vi "EngineSim.vi"() -> ()   [LabVIEW 2013]
uses:
  Typedefs/PWM.ctl
  <vilib>/NI/Engine Simulation Toolkit (EST)/APU/Settings.ctl
  <vilib>/NI/Engine Simulation Toolkit (EST)/APU/Input.ctl
  <vilib>/NI/Engine Simulation Toolkit (EST)/APU/Output.ctl
  <vilib>/NI/Engine Simulation Toolkit (EST)/ECU Event/Timing/Capture Output.ctl
  <vilib>/NI/Engine Simulation Toolkit (EST)/ECU Event/Timing/Measure Settings.ctl
  <vilib>/NI/Engine Simulation Toolkit (EST)/ECU Event/Timing/Measure Output.ctl
  <vilib>/NI/Engine Simulation Toolkit (EST)/Digital Pattern Generation/Settings.ctl
  <vilib>/NI/Engine Simulation Toolkit (EST)/Digital Pattern Generation/Input.ctl
  <vilib>/NI/Engine Simulation Toolkit (EST)/Digital Pattern Generation/Load Input.ctl
  <vilib>/NI/Engine Simulation Toolkit (EST)/Knock Sensor/Cylinder Input.ctl
  <vilib>/NI/Engine Simulation Toolkit (EST)/Knock Sensor/Cylinder Settings.ctl
  <vilib>/NI/Engine Simulation Toolkit (EST)/Knock Sensor/Generate Input.ctl
  <vilib>/NI/Engine Simulation Toolkit (EST)/Knock Sensor/Generate Settings.ctl
  <vilib>/NI/Engine Simulation Toolkit (EST)/Version Token.ctl
  <vilib>/NI/Engine Simulation Toolkit (EST)/APU/Shared Settings.ctl
  <vilib>/Platform/TimedLoop/XDataNode/timing_clust.ctl
  <vilib>/Platform/TimedLoop/XDataNode/nitl_modes.ctl
  <vilib>/Platform/TimedLoop/XDataNode/wakeup.ctl
  <vilib>/NI/Engine Simulation Toolkit (EST)/ECU Event/Timing/Capture Settings.ctl
  <vilib>/rvi/DataTransferAndStorage/Container/Common/niFpgaContainerGetUniqueNameForEmu.vi
  <vilib>/rvi/DataTransferAndStorage/Container/Common/niFpgaContainerSetEmuInfo.vi
  <vilib>/rvi/eio/common/nirviEmuReportErrorAndStop.vi
  <vilib>/rvi/Emulation/niFpgaSctlEmulationGetInTimedLoop.vi
  <vilib>/rvi/Emulation/niFpgaEmulationReportErrorSimple.vi
  <vilib>/rvi/Emulation/niFpgaGetClockAttributes.vi
  <vilib>/rvi/Emulation/niFpgaCriticalErrorInLSC.vi
  <vilib>/rvi/eio/common/nirviEmuTemplateMethod_errors.vi
  <vilib>/NI/Engine Simulation Toolkit (EST)/ECU Event/Timing/Measure Events (Non-40MHz).vi
  <vilib>/Platform/TimedLoop/XDataNode/XDataNode.xnode
  <vilib>/rvi/LocalResourceManager/LocalResourceManager.xnode
  <vilib>/eio/EIONode/EIONode.xnode
  <vilib>/Platform/TimedLoop/XDataNode/XDNodeRunTimeDep.lvlib
  <vilib>/NI/Engine Simulation Toolkit (EST)/APU/APU.lvlib
  <vilib>/NI/Engine Simulation Toolkit (EST)/ECU Event/Timing/ECU Event Timing.lvlib
  <vilib>/NI/Engine Simulation Toolkit (EST)/Digital Pattern Generation/Digital Pattern Generation.lvlib
  <vilib>/NI/Engine Simulation Toolkit (EST)/Knock Sensor/Knock Sensor.lvlib
  <vilib>/NI/Engine Simulation Toolkit (EST)/Engine Simulation Toolkit.lvlib
panel:
  in  "shared settings.apu":T1 {"cycle start" format="%#.15g"}
  in  "go.apu":bool
  in  "Spark Filter Ticks":fxp<+,11,11>=350.0
  in  "Injector Filter Ticks":fxp<+,11,11>=100.0
  in  "est.version":T2
  in  "settings.Knock AO 2":T3
  in  "settings.Knock AO 2.Cylinder 1":T4
  in  "settings.Knock AO 2.Cylinder 2":T4
  in  "settings.Knock AO 2.Cylinder 3":T4
  in  "settings.Knock AO 2.Cylinder 4":T4
  in  "input.Knock AO 2.Cylinder 1":T5
  in  "input.Knock AO 2.Cylinder 2":T5
  in  "input.Knock AO 2.Cylinder 3":T5
  in  "input.Knock AO 2.Cylinder 4":T5
  in  "input.Knock AO 2":T6
  in  "settings.Knock AO 2.Cylinder 5":T4
  in  "settings.Knock AO 2.Cylinder 6":T4
  in  "input.Knock AO 2.Cylinder 5":T5
  in  "input.Knock AO 2.Cylinder 6":T5
  in  "load input.Cam":T7
  in  "load input.Crank":T7
  in  "input.Crank":T8
  in  "settings.Crank":T9
  in  "input.Cam":T8
  in  "settings.Cam":T9
  out "status.Fuel6":T10
  in  "settings.Fuel6":T11
  out "capture.Fuel6.event 1":T12
  out "status.Fuel5":T10
  in  "settings.Fuel5":T11
  out "capture.Fuel5.event 1":T12
  out "status.Fuel4":T10
  in  "settings.Fuel4":T11
  out "capture.Fuel4.event 1":T12
  out "status.Fuel3":T10
  in  "settings.Fuel3":T11
  out "capture.Fuel3.event 1":T12
  out "status.Fuel2":T10
  in  "settings.Fuel2":T11
  out "capture.Fuel2.event 1":T12
  out "status.Fuel1":T10
  in  "settings.Fuel1":T11
  out "capture.Fuel1.event 1":T12
  out "status.Spark6":T10
  in  "settings.Spark6":T11
  out "capture.Spark6.event 1":T12
  out "status.Spark5":T10
  in  "settings.Spark5":T11
  out "capture.Spark5.event 1":T12
  out "status.Spark4":T10
  in  "settings.Spark4":T11
  out "capture.Spark4.event 1":T12
  out "status.Spark3":T10
  in  "settings.Spark3":T11
  out "capture.Spark3.event 1":T12
  out "status.Spark2":T10
  in  "settings.Spark2":T11
  out "capture.Spark2.event 1":T12
  out "status.Spark1":T10
  in  "settings.Spark1":T11
  out "capture.Spark1.event 1":T12
  out "output.apu":T13 caption="output"
  in  "input.apu":T14 caption="input"
  in  "settings.apu":T15
  in  "PWM write.Key Switch":T16
  in  "PWM write.Airflow":T16
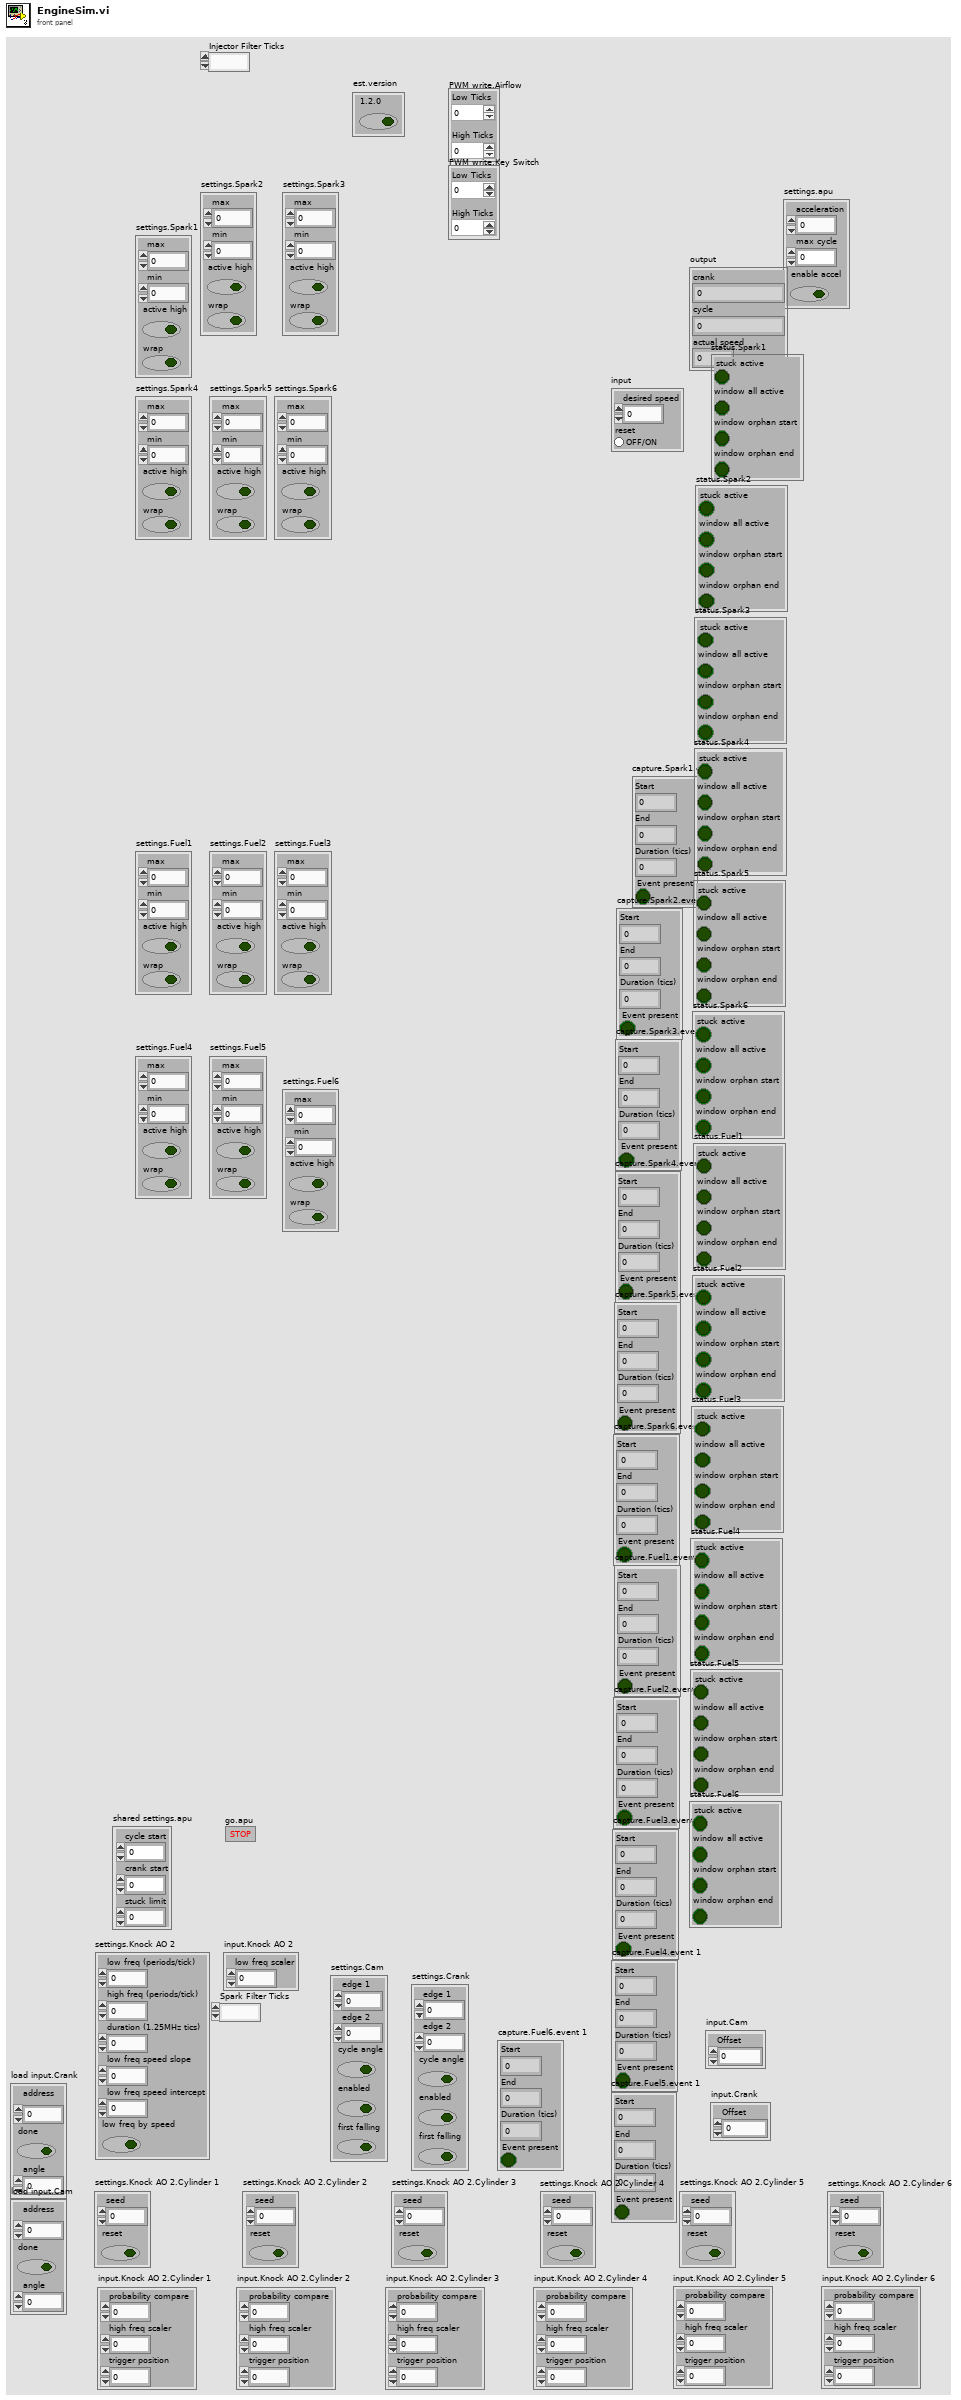
[diagram p1: front panel]
types:
  T1 = typedef "Engine Simulation Toolkit.lvlib/APU.lvlib/Shared Settings.ctl" = cluster{"cycle start":fxp<+,2,2>, "crank start":u16, "stuck limit":fxp<+,18,18>}
  T2 = typedef "Engine Simulation Toolkit.lvlib/Version Token.ctl" = cluster{"1.2.0":bool}
  T3 = typedef "Engine Simulation Toolkit.lvlib/Knock Sensor.lvlib/Generate Settings.ctl" = cluster{"low freq (periods/tick)":fxp<+,32,0>, "high freq (periods/tick)":fxp<+,32,0>, "duration (1.25MHz tics)":fxp<+,18,18>, "low freq speed slope":fxp<+,16,-3>, "low freq speed intercept":fxp<+,10,-10>, "low freq by speed":bool}
  T4 = typedef "Engine Simulation Toolkit.lvlib/Knock Sensor.lvlib/Cylinder Settings.ctl" = cluster{"seed":u16, "reset":bool}
  T5 = typedef "Engine Simulation Toolkit.lvlib/Knock Sensor.lvlib/Cylinder Input.ctl" = cluster{"probability compare":u16, "high freq scaler":fxp<+,10,0>, "trigger position":u16}
  T6 = typedef "Engine Simulation Toolkit.lvlib/Knock Sensor.lvlib/Generate Input.ctl" = cluster{"low freq scaler":fxp<+,10,0>}
  T7 = typedef "Engine Simulation Toolkit.lvlib/Digital Pattern Generation.lvlib/Load Input.ctl" = cluster{"address":fxp<+,11,11>, "done":bool, "angle":u16}
  T8 = typedef "Engine Simulation Toolkit.lvlib/Digital Pattern Generation.lvlib/Input.ctl" = cluster{"Offset":i16}
  T9 = typedef "Engine Simulation Toolkit.lvlib/Digital Pattern Generation.lvlib/Settings.ctl" = cluster{"edge 1":u16, "edge 2":u16, "cycle angle":bool, "enabled":bool, "first falling":bool}
  T10 = typedef "Engine Simulation Toolkit.lvlib/ECU Event Timing.lvlib/Measure Output.ctl" = cluster{"stuck active":bool, "window all active":bool, "window orphan start":bool, "window orphan end":bool}
  T11 = typedef "Engine Simulation Toolkit.lvlib/ECU Event Timing.lvlib/Measure Settings.ctl" = cluster{"max":u16, "min":u16, "active high":bool, "wrap":bool}
  T12 = typedef "Engine Simulation Toolkit.lvlib/ECU Event Timing.lvlib/Capture Output.ctl" = cluster{"Start":u16, "End":u16, "Duration (tics)":fxp<+,18,18>, "Event present":bool}
  T13 = typedef "Engine Simulation Toolkit.lvlib/APU.lvlib/Output.ctl" = cluster{"crank":u16, "cycle":u16, "actual speed":fxp<+/-,23,2>}
  T14 = typedef "Engine Simulation Toolkit.lvlib/APU.lvlib/Input.ctl" = cluster{"desired speed":fxp<+/-,23,2>, "reset":bool}
  T15 = typedef "Engine Simulation Toolkit.lvlib/APU.lvlib/Settings.ctl" = cluster{"acceleration":fxp<+,18,-20>, "max cycle":fxp<+,2,2>, "enable accel":bool}
  T16 = typedef "PWM.ctl" = cluster{"Low Ticks":u32, "High Ticks":u32}
  T17 = typedef "XDNodeRunTimeDep.lvlib/timing_clust.ctl" = cluster{"Expected End [f-1]":u64, "Actual End [f-1]":u64, "Finished Late? [f-1]":bool, "Expected End [i-1]":u64, "Actual End [i-1]":u64, "Finished Late? [i-1]":bool, "Expected Start [i]":u64, "Actual Start [i]":u64, "Expected Start [f]":u64, "Actual Start [f]":u64, "Source Name":string, "Structure Name":string, "Period":i64, "Deadline":i64, "Offset":i64, "Start":i64, "Priority":i32, "Timeout":i32, "Mode":T18, "Wakeup Reason":T19, "Error":errorcluster, "Source Type":string, "Secondary Source Type":string, "Global End Time":u64, "Global Start Time":u64, "Frame Duration":u64, "Iteration Duration":u64, "Assigned CPU":i32, "I/O Scan Engine Mode":u32}
  T18 = typedef "XDNodeRunTimeDep.lvlib/nitl_modes.ctl" = enum32{"No Change", "Process missed periods, maintain original phase", "Discard missed periods, maintain original phase", "Process missed periods, ignore original phase", "Discard missed periods, ignore original phase"}
  T19 = typedef "XDNodeRunTimeDep.lvlib/wakeup.ctl" = enum32{"Normal", "Aborted", "Asynchronous wakeup", "Timing source error", "Timed loop error", "Timeout"}
  T20 = typedef "Engine Simulation Toolkit.lvlib/Digital Pattern Generation.lvlib/Load Data.ctl" = cluster{"max address":fxp<+,11,11>, "memory":refnum<k21>}
  T21 = typedef "Engine Simulation Toolkit.lvlib/APU.lvlib/Register Bus.ctl" = cluster{"Speed":refnum<k21>, "Crank Angle":refnum<k21>, "Cycle Angle":refnum<k21>, "Crank Count":refnum<k21>, "Cycle Count":refnum<k21>, "1.25 MHz Counter":refnum<k21>, "shared settings":T1}
  T22 = typedef "Engine Simulation Toolkit.lvlib/ECU Event Timing.lvlib/Capture Settings.ctl" = u8
  T23 = typedef "Engine Simulation Toolkit.lvlib/ECU Event Timing.lvlib/Measured Data.ctl" = cluster{"start":u16, "end":u16, "duration (tics)":fxp<+,18,18>, "window end":bool, "window begin":bool, "pulse end":bool, "pulse #":u8}
  T24 = typedef "Engine Simulation Toolkit.lvlib/Knock Sensor.lvlib/Triggered Cylinder Data.ctl" = cluster{"trigger knock":bool, "high freq scaler":fxp<+,10,0>}
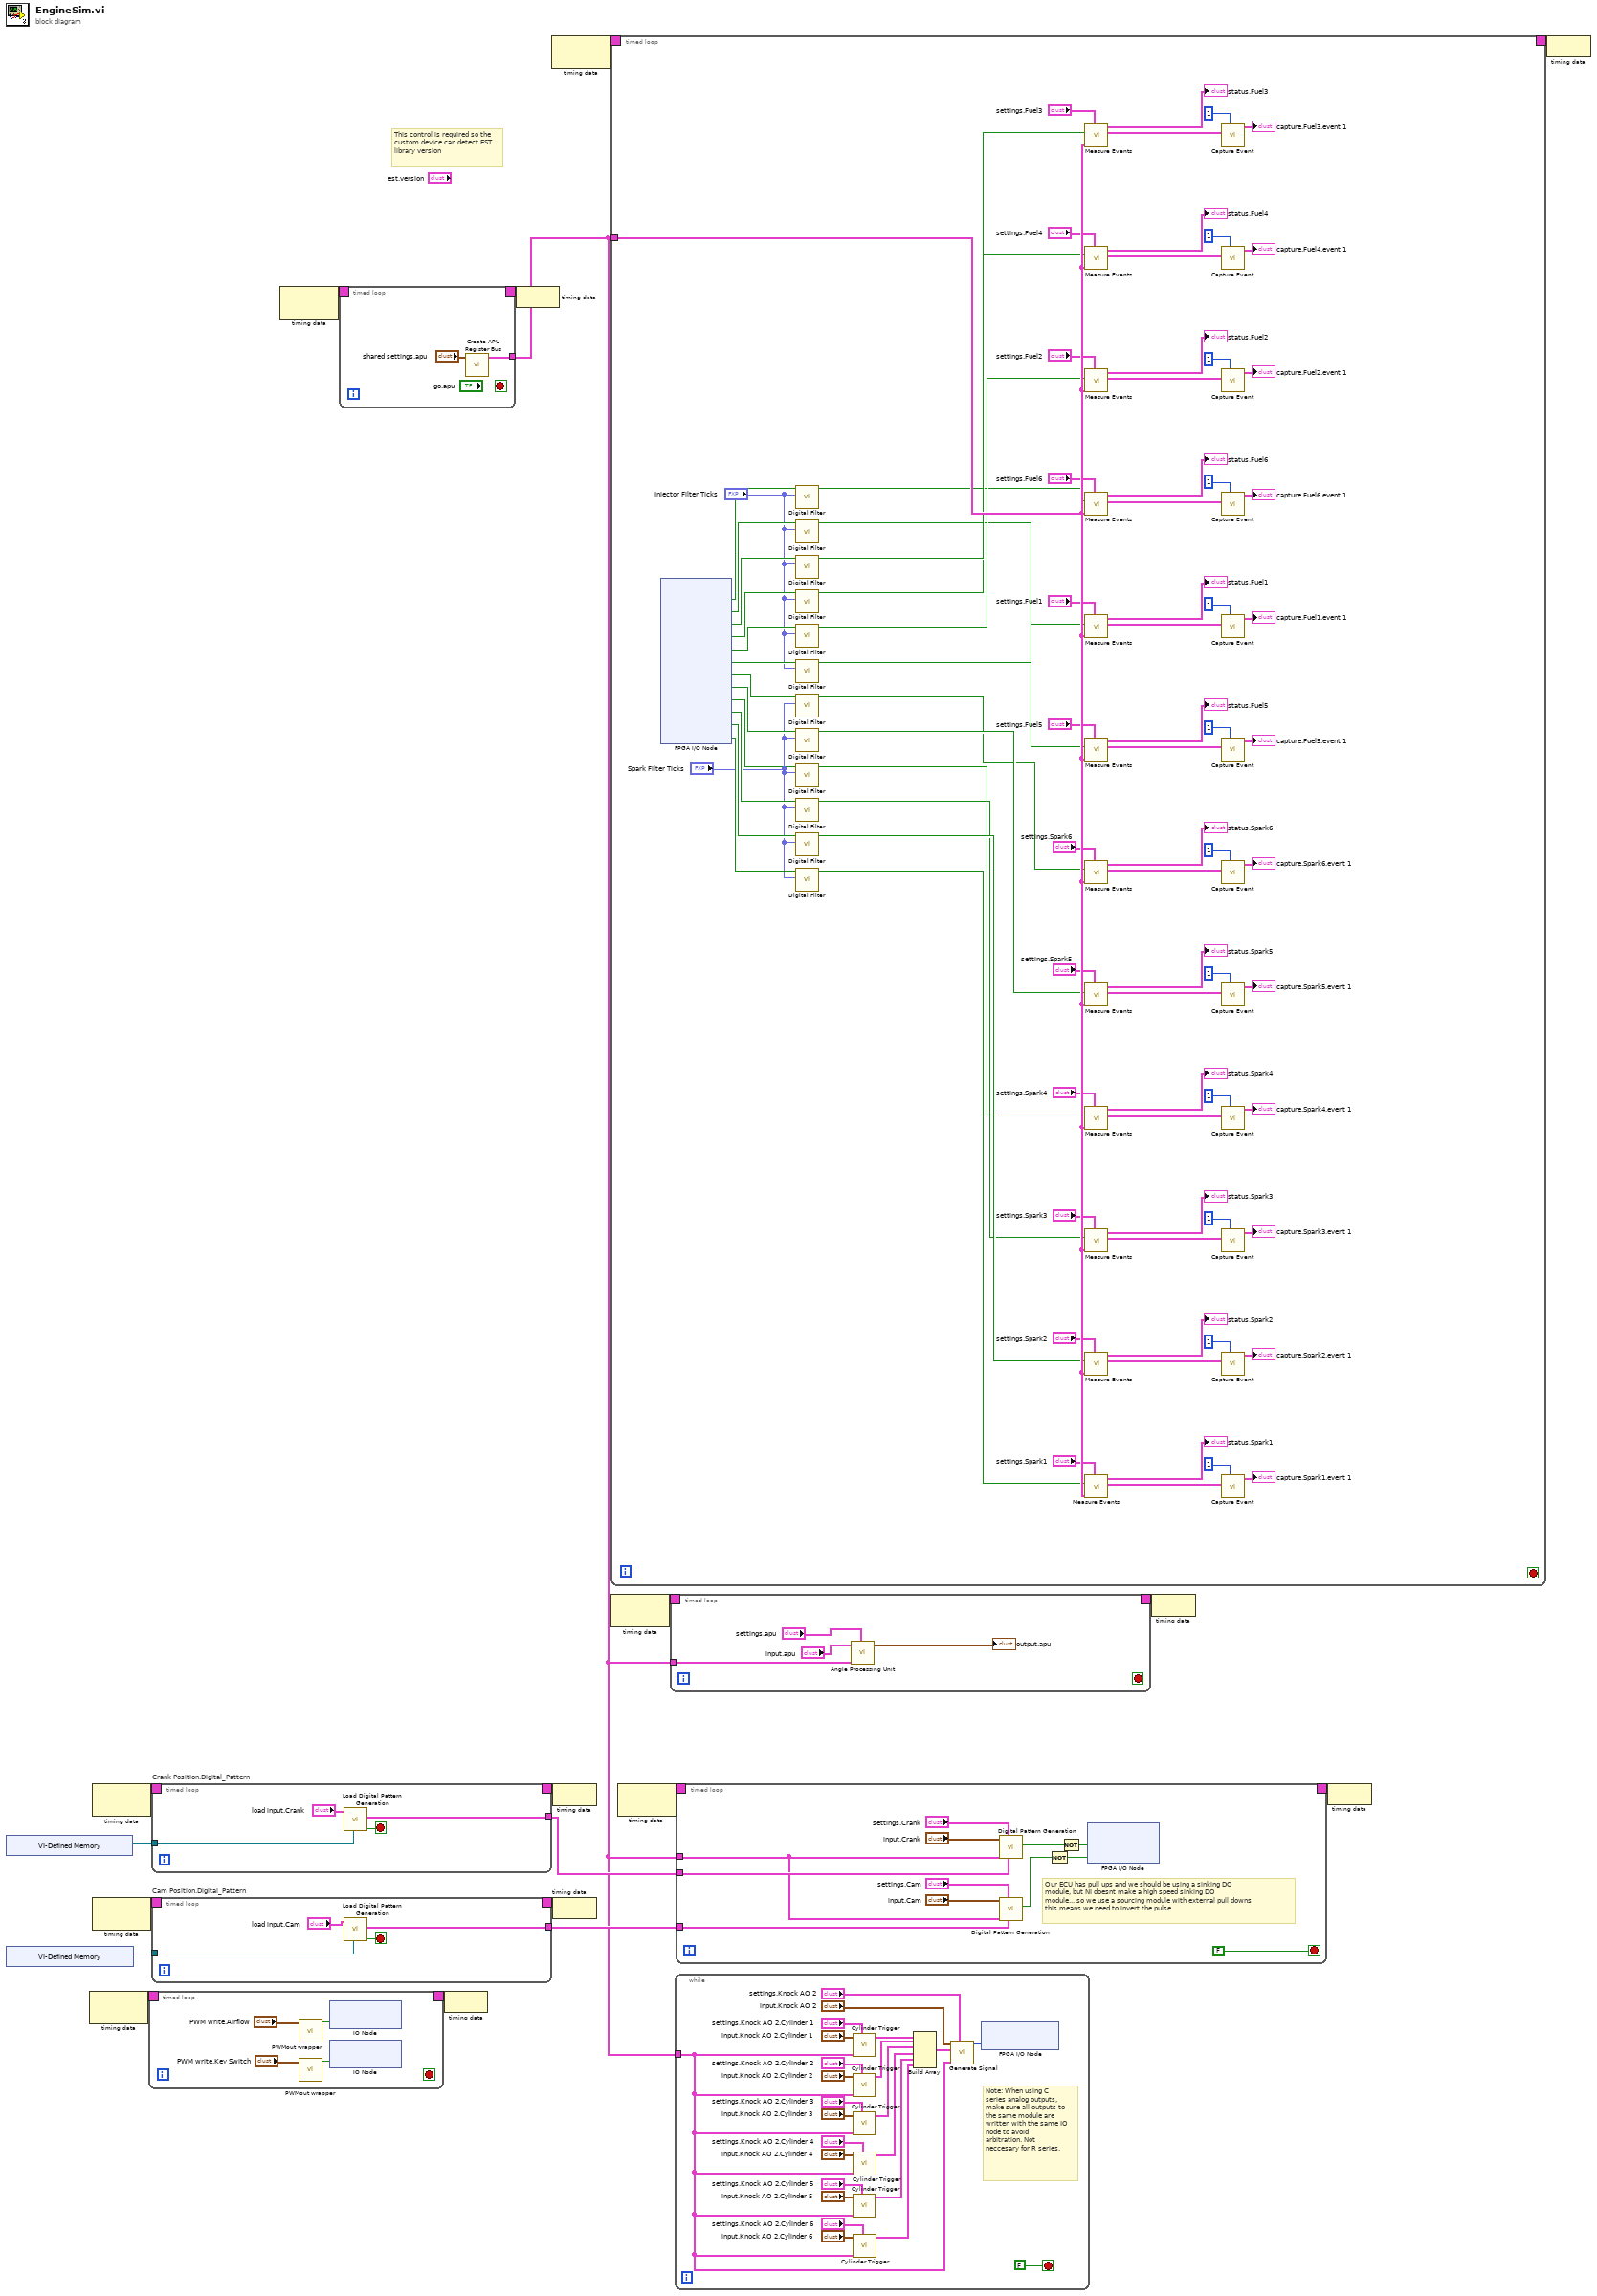
[diagram p0: block diagram]
diagram:
  # "This control is required so the custom device can detect EST library version"
  n1 = xnode "VI-Defined Memory"() -> ("Memory Out"=w7:refnum<k21>)
  n2 = xnode "VI-Defined Memory"() -> ("Memory Out"=w6:refnum<k21>)
  n3 = node-c288() -> (w19:T17)  [unwired: 1 in]
  n4 = node-c288() -> (w13:T17)  [unwired: 1 in]
  n5 = node-c288() -> (w11:T17)  [unwired: 1 in]
  n6 = timed-loop {
    timing: w19 -> [_]
    timing-out: [_] -> w18
    stop <- _ stop-if-true
    n7 = call "PWMout wrapper.vi"("PWM in"="PWM write.Airflow") -> ("Value"=w23:bool)  [unwired: 10 in]
    n8 = call "PWMout wrapper.vi"("PWM in"="PWM write.Key Switch") -> ("Value"=w21:bool)  [unwired: 10 in]
    n9 = xnode ("IO Node")("9474/DO3"=w23) -> ()  [unwired: 1 in, 1 out]
    n10 = xnode ("IO Node")("9474/DO4"=w21) -> ()  [unwired: 1 in, 1 out]
  }
  n11 = timed-loop "Crank Position.Digital_Pattern" {
    timing: w13 -> [_]
    timing-out: [_] -> w12
    tunnel: w7 -> [w28]
    tunnel: [w27] -> w9
    stop <- w29 stop-if-true
    n12 = call <vilib>:"Load Digital Pattern Generation.vi"("memory"=w28, "load input.<user name>"="load input.Crank") -> ("done"=w29:bool, "load data"=w27:T20)  [unwired: 8 in]
  }
  n13 = timed-loop "Cam Position.Digital_Pattern" {
    timing: w11 -> [_]
    timing-out: [_] -> w10
    tunnel: w6 -> [w34]
    tunnel: [w33] -> w8
    stop <- w35 stop-if-true
    n14 = call <vilib>:"Load Digital Pattern Generation.vi"("memory"=w34, "load input.<user name>"="load input.Cam") -> ("done"=w35:bool, "load data"=w33:T20)  [unwired: 8 in]
  }
  n15 = node-c288() -> (w3:T17)  [unwired: 1 in]
  n16 = timed-loop {
    timing: w3 -> [_]
    timing-out: [_] -> w2
    tunnel: [w39] -> w1
    stop <- "go.apu" stop-if-true
    n17 = call <vilib>:"Create APU Register Bus.vi"("shared settings.<user name>"="shared settings.apu") -> ("register bus"=w39:T21)  [unwired: 10 in]
  }
  n18 = node-c288(w18) -> ()
  n19 = node-c288(w2) -> ()
  n20 = node-c288() -> (w5:T17)  [unwired: 1 in]
  n21 = node-c288(w12) -> ()
  n22 = node-c288(w10) -> ()
  n23 = timed-loop "NI 9403" {
    tunnel: w1 -> [w129]
    timing: w5 -> [_]
    timing-out: [_] -> w4
    stop <- _ stop-if-true
    n24 = xnode "FPGA I/O Node"() -> ("Fuel/DI5"=w128:bool, "Fuel/DI4"=w127:bool, "Fuel/DI3"=w126:bool, "Fuel/DI2"=w125:bool, "Fuel/DI1"=w124:bool, "Fuel/DI0"=w123:bool, "Spark/DI5"=w122:bool, "Spark/DI4"=w121:bool, "Spark/DI3"=w120:bool, "Spark/DI2"=w119:bool, "Spark/DI1"=w118:bool, "Spark/DI0"=w117:bool)  [unwired: 12 in, 12 out]
    n25 = call "Digital Filter.vi"("Tics to Filter"="Injector Filter Ticks", "Input Signal"=w128) -> ("Output Filtered Signal"=w48:bool)  [unwired: 9 in]
    n26 = call "Digital Filter.vi"("Tics to Filter"="Injector Filter Ticks", "Input Signal"=w127) -> ("Output Filtered Signal"=w49:bool)  [unwired: 9 in]
    n27 = call "Digital Filter.vi"("Tics to Filter"="Injector Filter Ticks", "Input Signal"=w126) -> ("Output Filtered Signal"=w50:bool)  [unwired: 9 in]
    n28 = call "Digital Filter.vi"("Tics to Filter"="Injector Filter Ticks", "Input Signal"=w125) -> ("Output Filtered Signal"=w45:bool)  [unwired: 9 in]
    n29 = call "Digital Filter.vi"("Tics to Filter"="Injector Filter Ticks", "Input Signal"=w124) -> ("Output Filtered Signal"=w51:bool)  [unwired: 9 in]
    n30 = call "Digital Filter.vi"("Tics to Filter"="Injector Filter Ticks", "Input Signal"=w123) -> ("Output Filtered Signal"=w52:bool)  [unwired: 9 in]
    n31 = call "Digital Filter.vi"("Tics to Filter"="Spark Filter Ticks", "Input Signal"=w122) -> ("Output Filtered Signal"=w53:bool)  [unwired: 9 in]
    n32 = call "Digital Filter.vi"("Tics to Filter"="Spark Filter Ticks", "Input Signal"=w121) -> ("Output Filtered Signal"=w54:bool)  [unwired: 9 in]
    n33 = call "Digital Filter.vi"("Tics to Filter"="Spark Filter Ticks", "Input Signal"=w120) -> ("Output Filtered Signal"=w47:bool)  [unwired: 9 in]
    n34 = call "Digital Filter.vi"("Tics to Filter"="Spark Filter Ticks", "Input Signal"=w119) -> ("Output Filtered Signal"=w55:bool)  [unwired: 9 in]
    n35 = call "Digital Filter.vi"("Tics to Filter"="Spark Filter Ticks", "Input Signal"=w118) -> ("Output Filtered Signal"=w56:bool)  [unwired: 9 in]
    n36 = call "Digital Filter.vi"("Tics to Filter"="Spark Filter Ticks", "Input Signal"=w117) -> ("Output Filtered Signal"=w46:bool)  [unwired: 9 in]
    n37 = call-poly <vilib>:"Measure Events.vi"("settings.<user name>"="settings.Fuel3", "register bus"=w129, "event"=w45) -> ("measured data"=w73:T23, "status.<user name>"=→"status.Fuel3":T10)  [unwired: 7 in]
    n38 = call-poly <vilib>:"Measure Events.vi"("settings.<user name>"="settings.Fuel4", "register bus"=w129, "event"=w50) -> ("measured data"=w68:T23, "status.<user name>"=→"status.Fuel4":T10)  [unwired: 7 in]
    n39 = call-poly <vilib>:"Measure Events.vi"("settings.<user name>"="settings.Fuel2", "register bus"=w129, "event"=w51) -> ("measured data"=w78:T23, "status.<user name>"=→"status.Fuel2":T10)  [unwired: 7 in]
    n40 = call-poly <vilib>:"Measure Events.vi"("settings.<user name>"="settings.Fuel6", "register bus"=w129, "event"=w48) -> ("measured data"=w58:T23, "status.<user name>"=→"status.Fuel6":T10)  [unwired: 7 in]
    n41 = call-poly <vilib>:"Measure Events.vi"("settings.<user name>"="settings.Fuel1", "register bus"=w129, "event"=w52) -> ("measured data"=w83:T23, "status.<user name>"=→"status.Fuel1":T10)  [unwired: 7 in]
    n42 = call-poly <vilib>:"Measure Events.vi"("settings.<user name>"="settings.Fuel5", "register bus"=w129, "event"=w49) -> ("measured data"=w63:T23, "status.<user name>"=→"status.Fuel5":T10)  [unwired: 7 in]
    n43 = call-poly <vilib>:"Measure Events.vi"("settings.<user name>"="settings.Spark6", "register bus"=w129, "event"=w53) -> ("measured data"=w88:T23, "status.<user name>"=→"status.Spark6":T10)  [unwired: 7 in]
    n44 = call-poly <vilib>:"Measure Events.vi"("settings.<user name>"="settings.Spark5", "register bus"=w129, "event"=w54) -> ("measured data"=w93:T23, "status.<user name>"=→"status.Spark5":T10)  [unwired: 7 in]
    n45 = call-poly <vilib>:"Measure Events.vi"("settings.<user name>"="settings.Spark4", "register bus"=w129, "event"=w47) -> ("measured data"=w98:T23, "status.<user name>"=→"status.Spark4":T10)  [unwired: 7 in]
    n46 = call-poly <vilib>:"Measure Events.vi"("settings.<user name>"="settings.Spark3", "register bus"=w129, "event"=w55) -> ("measured data"=w103:T23, "status.<user name>"=→"status.Spark3":T10)  [unwired: 7 in]
    n47 = call-poly <vilib>:"Measure Events.vi"("settings.<user name>"="settings.Spark2", "register bus"=w129, "event"=w56) -> ("measured data"=w108:T23, "status.<user name>"=→"status.Spark2":T10)  [unwired: 7 in]
    n48 = call-poly <vilib>:"Measure Events.vi"("settings.<user name>"="settings.Spark1", "register bus"=w129, "event"=w46) -> ("measured data"=w113:T23, "status.<user name>"=→"status.Spark1":T10)  [unwired: 7 in]
    n49 = call <vilib>:"Capture Event.vi"("event # to capture"=T22 1 ("Settings.spark 1 shot 1"), "measured data"=w73) -> ("capture.<user name>"=→"capture.Fuel3.event 1":T12)  [unwired: 9 in]
    n50 = call <vilib>:"Capture Event.vi"("event # to capture"=T22 1 ("Settings.spark 1 shot 1"), "measured data"=w68) -> ("capture.<user name>"=→"capture.Fuel4.event 1":T12)  [unwired: 9 in]
    n51 = call <vilib>:"Capture Event.vi"("event # to capture"=T22 1 ("Settings.spark 1 shot 1"), "measured data"=w78) -> ("capture.<user name>"=→"capture.Fuel2.event 1":T12)  [unwired: 9 in]
    n52 = call <vilib>:"Capture Event.vi"("event # to capture"=T22 1 ("Settings.spark 1 shot 1"), "measured data"=w58) -> ("capture.<user name>"=→"capture.Fuel6.event 1":T12)  [unwired: 9 in]
    n53 = call <vilib>:"Capture Event.vi"("event # to capture"=T22 1 ("Settings.spark 1 shot 1"), "measured data"=w83) -> ("capture.<user name>"=→"capture.Fuel1.event 1":T12)  [unwired: 9 in]
    n54 = call <vilib>:"Capture Event.vi"("event # to capture"=T22 1 ("Settings.spark 1 shot 1"), "measured data"=w63) -> ("capture.<user name>"=→"capture.Fuel5.event 1":T12)  [unwired: 9 in]
    n55 = call <vilib>:"Capture Event.vi"("event # to capture"=T22 1 ("Settings.spark 1 shot 1"), "measured data"=w88) -> ("capture.<user name>"=→"capture.Spark6.event 1":T12)  [unwired: 9 in]
    n56 = call <vilib>:"Capture Event.vi"("event # to capture"=T22 1 ("Settings.spark 1 shot 1"), "measured data"=w93) -> ("capture.<user name>"=→"capture.Spark5.event 1":T12)  [unwired: 9 in]
    n57 = call <vilib>:"Capture Event.vi"("event # to capture"=T22 1 ("Settings.spark 1 shot 1"), "measured data"=w98) -> ("capture.<user name>"=→"capture.Spark4.event 1":T12)  [unwired: 9 in]
    n58 = call <vilib>:"Capture Event.vi"("event # to capture"=T22 1 ("Settings.spark 1 shot 1"), "measured data"=w103) -> ("capture.<user name>"=→"capture.Spark3.event 1":T12)  [unwired: 9 in]
    n59 = call <vilib>:"Capture Event.vi"("event # to capture"=T22 1 ("Settings.spark 1 shot 1"), "measured data"=w108) -> ("capture.<user name>"=→"capture.Spark2.event 1":T12)  [unwired: 9 in]
    n60 = call <vilib>:"Capture Event.vi"("event # to capture"=T22 1 ("Settings.spark 1 shot 1"), "measured data"=w113) -> ("capture.<user name>"=→"capture.Spark1.event 1":T12)  [unwired: 9 in]
  }
  n61 = node-c288() -> (w17:T17)  [unwired: 1 in]
  n62 = node-c288() -> (w15:T17)  [unwired: 1 in]
  n63 = timed-loop {
    timing: w17 -> [_]
    timing-out: [_] -> w16
    tunnel: w1 -> [w133]
    stop <- _ stop-if-true
    n64 = call <vilib>:"Angle Processing Unit.vi"("settings.<user name>"="settings.apu", "register bus"=w133, "input.<user name>"="input.apu") -> ("output.<user name>"=→"output.apu":T13)  [unwired: 8 in]
  }
  n65 = while {
    tunnel: w1 -> [w138]
    stop <- FALSE stop-if-true
    # "Note: When using C series analog outputs, make sure all outputs to the same module are written with the same IO node to avoid arbitration. Not neccesary for R series."
    n66 = call <vilib>:"Cylinder Trigger.vi"("settings.<user name>"="settings.Knock AO 2.Cylinder 1", "register bus"=w138, "input.<user name>"="input.Knock AO 2.Cylinder 1") -> ("triggered knock data"=w161:T24)  [unwired: 8 in]
    n67 = call <vilib>:"Cylinder Trigger.vi"("settings.<user name>"="settings.Knock AO 2.Cylinder 2", "register bus"=w138, "input.<user name>"="input.Knock AO 2.Cylinder 2") -> ("triggered knock data"=w160:T24)  [unwired: 8 in]
    n68 = call <vilib>:"Cylinder Trigger.vi"("settings.<user name>"="settings.Knock AO 2.Cylinder 3", "register bus"=w138, "input.<user name>"="input.Knock AO 2.Cylinder 3") -> ("triggered knock data"=w159:T24)  [unwired: 8 in]
    n69 = call <vilib>:"Cylinder Trigger.vi"("settings.<user name>"="settings.Knock AO 2.Cylinder 5", "register bus"=w138, "input.<user name>"="input.Knock AO 2.Cylinder 5") -> ("triggered knock data"=w140:T24)  [unwired: 8 in]
    n70 = call <vilib>:"Cylinder Trigger.vi"("settings.<user name>"="settings.Knock AO 2.Cylinder 4", "register bus"=w138, "input.<user name>"="input.Knock AO 2.Cylinder 4") -> ("triggered knock data"=w158:T24)  [unwired: 8 in]
    n71 = call <vilib>:"Cylinder Trigger.vi"("settings.<user name>"="settings.Knock AO 2.Cylinder 6", "register bus"=w138, "input.<user name>"="input.Knock AO 2.Cylinder 6") -> ("triggered knock data"=w139:T24)  [unwired: 8 in]
    n72 = Build Array(w161, w160, w159, w158, w140, w139) -> (w157:T24[])
    n73 = call <vilib>:"Generate Signal.vi"("settings.<user name>"="settings.Knock AO 2", "register bus"=w138, "triggered knock data"=w157, "input.<user name>"="input.Knock AO 2") -> ("knock signal"=w145:i16)  [unwired: 7 in]
    n74 = xnode ("FPGA I/O Node")("Knock/AO0"=w145) -> ()  [unwired: 1 in, 1 out]
  }
  n75 = timed-loop "Timed Loop" {
    timing: w15 -> [_]
    timing-out: [_] -> w14
    tunnel: w8 -> [w166]
    tunnel: w9 -> [w165]
    tunnel: w1 -> [w164]
    stop <- FALSE stop-if-true
    # "Our ECU has pull ups and we should be using a sinking DO\nmodule, but NI doesnt make a high speed sinking DO\nmodule... so we use a sourcing module with external pull downs\nthis means we need to invert the pulse"
    n76 = call <vilib>:"Digital Pattern Generation.vi"("load data"=w165, "settings.<user name>"="settings.Crank", "register bus"=w164, "input.<user name>"="input.Crank") -> ("digial output"=w170:bool)  [unwired: 7 in]
    n77 = call <vilib>:"Digital Pattern Generation.vi"("load data"=w166, "settings.<user name>"="settings.Cam", "register bus"=w164, "input.<user name>"="input.Cam") -> ("digial output"=w167:bool)  [unwired: 7 in]
    n78 = Not(x=w167) -> (.not. x?=w162:bool)
    n79 = Not(x=w170) -> (.not. x?=w163:bool)
    n80 = xnode ("FPGA I/O Node")("9474/DO0"=w163, "9474/DO1"=w162) -> ()  [unwired: 2 in, 2 out]
  }
  n81 = node-c288(w16) -> ()
  n82 = node-c288(w14) -> ()
  n83 = node-c288(w4) -> ()
